vi "Check for Marker.vi"(8 "error in (no error)":errorcluster, 11 "Mouse in":refnum<class "Mouse.lvclass">) -> (0 "error out":errorcluster, 2 "Marker Present?":bool, 3 "Mouse out":refnum<class "Mouse.lvclass">)   [LabVIEW 2020, in "Maze.lvlib" / "Mouse.lvclass"]
doc: "Checks to see if a marker has been placed on the floor. Markers can be dropped or picked up to facilitate algorithms that need to keep track of where they've been and don't want to try and build their own internal map. Using markers will score lower as it means an internal map is not being built within the mouse implementation."
uses:
  Mouse.lvclass
  Mouse.lvclass/Mouse.ctl
  Maze/Maze.lvclass
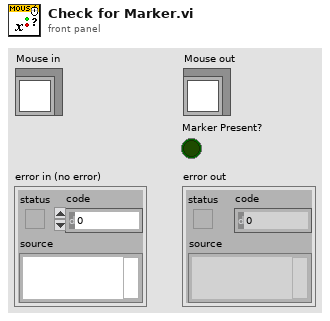
[diagram p1: front panel]
types:
  T1 = typedef "Maze.lvlib/Position.ctl" = cluster{"S":i32, "E":i32}
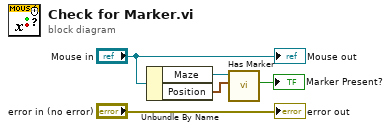
[diagram p0: block diagram]
diagram:
  n1 = Unbundle By Name("Mouse in") -> ("Maze"=w3:refnum<class "Maze.lvclass">, "Position"=w2:T1)
  n2 = call "Has Marker.vi"("Position"=w2, "Maze in"=w3) -> ("Has Marker?"=→"Marker Present?":bool)  [unwired: 7 in, 2 out]
  "error out" <- "error in (no error)"
  "Mouse out" <- "Mouse in"
